vi "Read Jitter Measurement.vi"   [LabVIEW 2015, in "Agilent 2000 3000 X-Series.lvlib"]
doc: "Read Jitter Measurement Polymorphic VI"
uses:
  <instrlib>/Agilent 2000 3000 X-Series/Agilent 2000 3000 X-Series.lvlib
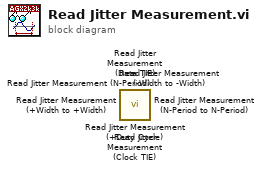
[diagram p0: block diagram]
diagram:
  n1 = call <instrlib>:"Read Jitter Measurement (+Duty Cycle).vi"() -> ()  [unwired: 9 in, 3 out]
  n2 = call <instrlib>:"Read Jitter Measurement (-Width to -Width).vi"() -> ()  [unwired: 9 in, 3 out]
  n3 = call <instrlib>:"Read Jitter Measurement (+Width to +Width).vi"() -> ()  [unwired: 9 in, 3 out]
  n4 = call <instrlib>:"Read Jitter Measurement (N-Period to N-Period).vi"() -> ()  [unwired: 9 in, 3 out]
  n5 = call <instrlib>:"Read Jitter Measurement (N-Period).vi"() -> ()  [unwired: 9 in, 3 out]
  n6 = call <instrlib>:"Read Jitter Measurement (Data TIE).vi"() -> ()  [unwired: 9 in, 3 out]
  n7 = call <instrlib>:"Read Jitter Measurement (Clock TIE).vi"() -> ()  [unwired: 9 in, 3 out]
